vi "Get_API_Mode.vi"(1 "Argument List":string[](array[string])) -> (0 "API Mode":T1(ring))   [LabVIEW 2011]
doc: "This VI returns the API mode determined by the \"Argument List\" parameter. See Set_API_Mode.vi for a complete description of the various API modes."
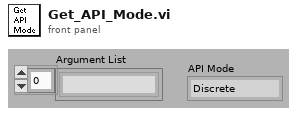
[diagram p1: front panel]
types:
  T1 = enum16{"Discrete", "Continuous", "Instantaneous", "Finite"}
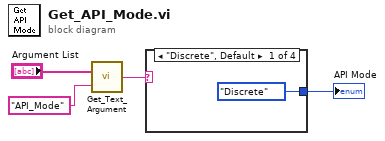
[diagram p0: block diagram]
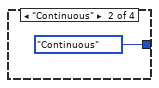
[diagram p2: hidden frame]
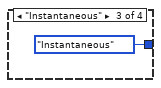
[diagram p3: hidden frame]
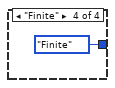
[diagram p4: hidden frame]
diagram:
  n1 = call "Get_Text_Argument.vi"("Argument"="API_Mode", "Argument List"="Argument List") -> ("Text"=w3:string)
  n2 = case shown="\"Discrete\", Default" w3 {
    tunnel: [T1."Discrete" ("API Mode") T1."Continuous" ("API Mode") T1."Instantaneous" ("API Mode") T1."Finite" ("API Mode")] -> w1
    frame "Discrete", Default {
    }
    frame "Continuous" {
    }
    frame "Instantaneous" {
    }
    frame "Finite" {
    }
  }
  "API Mode" <- w1
